vi "Pixel Sclera Check.vi"(9 "Blue":sgl, 10 "Green":sgl, 11 "Red":sgl) -> (3 "RGB Sclera":bool)   [LabVIEW 2015]
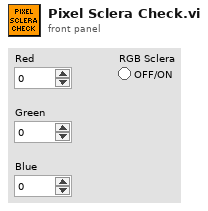
[diagram p1: front panel]
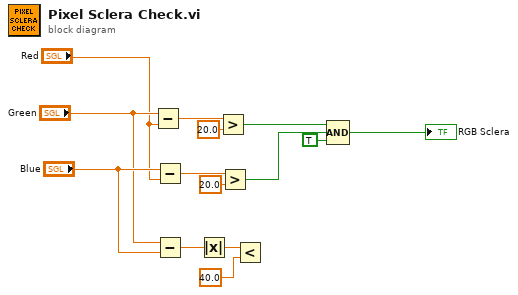
[diagram p0: block diagram]
diagram:
  n1 = Subtract(x="Green", y="Red") -> (x-y=w2:sgl)
  n2 = Subtract(x="Blue", y="Red") -> (x-y=w5:sgl)
  n3 = Subtract(x="Green", y="Blue") -> (x-y=w9:sgl)
  n4 = Absolute Value(x=w9) -> (abs(x)=w10:sgl)
  n5 = Greater?(x=w2, y=sgl 20.0) -> (0:w12:bool)
  n6 = Greater?(x=w5, y=sgl 20.0) -> (0:w13:bool)
  n7 = Less?(x=w10, y=sgl 40.0) -> ()  [unwired: 1 out]
  n8 = Compound Arithmetic op=AND(w12, w13, TRUE ("value")) -> (→"RGB Sclera":bool)
